vi "Periodic Dot Tracking.vi"() -> ()   [LabVIEW 2012]
panel:
  in  "Delay Time (s)":dbl=1.0
  in  "stop":bool
  out "Gave up?":bool
  out "Y Gauss Amplitude":dbl
  out "Cross Section Y":dbl[](graph)
  out "Cross Section X":dbl[](graph)
  out "Z Position":dbl
  out "Y Position":dbl
  out "X Position":dbl
  in  "Z-track?":bool=TRUE
  in  "Z Pos":dbl=52.1
  in  "Y pos":dbl=35.0
  in  "X Pos":dbl=192.0
  in  "Y Parameters":T1={"Number of Y Steps"=200, "Max Y (V)"=1.0, "Min Y (V)"=-1.0}
  in  "X Parameters":T2={"Number of X Steps"=200, "Max X (V)"=1.0, "Min X (V)"=-1.0}
  in  "RS232 settings":cluster{"Portnumber":i32, "Baudrate":u16}={"Portnumber"=12, "Baudrate"=5} {"Portnumber" items=["COM1", "COM2", "COM3", "COM4", "COM5", "COM6", "COM7", "COM8", "COM9", "COM10", "COM11", "COM12", "COM13", "COM14", "COM15", "COM16", "COM17", "COM18", "COM19", "COM20", "COM21", "COM22", "COM23", "COM24", "COM25", "COM26", "COM27", "COM28", "COM29", "COM30"]; "Baudrate" items=["9600", "14400", "19200", "38400", "57600", "115200"]}
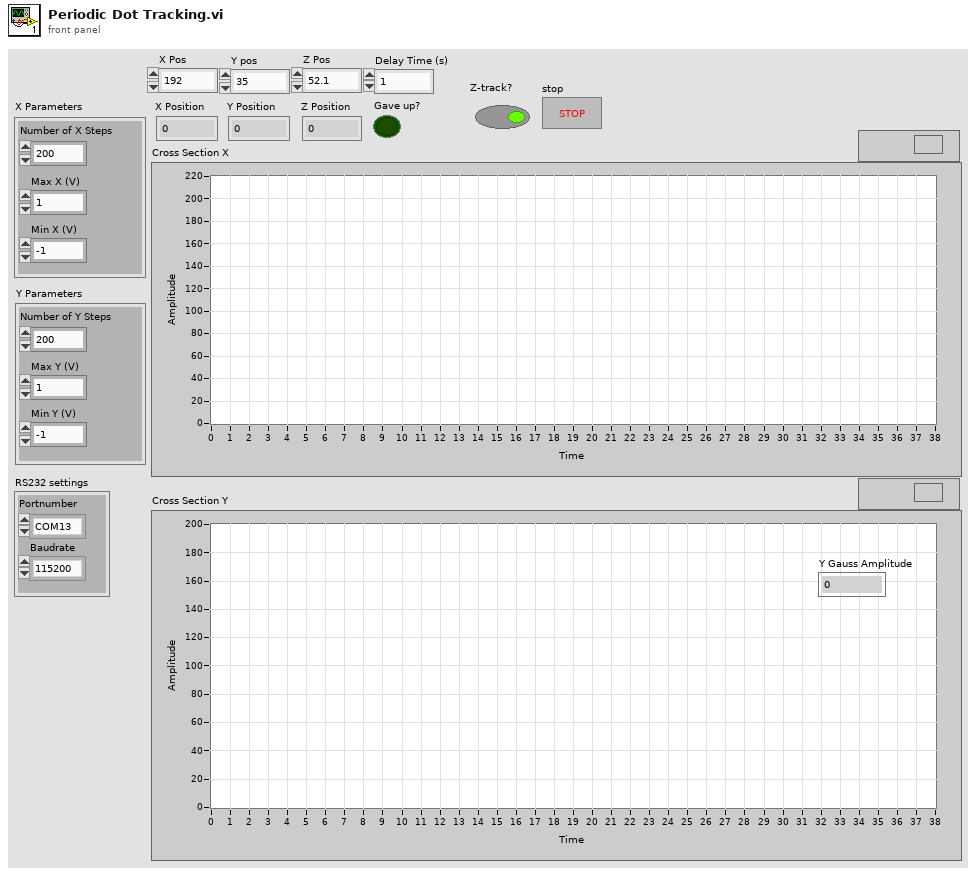
[diagram p1: front panel]
types:
  T1 = cluster{"Number of Y Steps":i32, "Max Y (V)":dbl, "Min Y (V)":dbl}
  T2 = cluster{"Number of X Steps":i32, "Max X (V)":dbl, "Min X (V)":dbl}
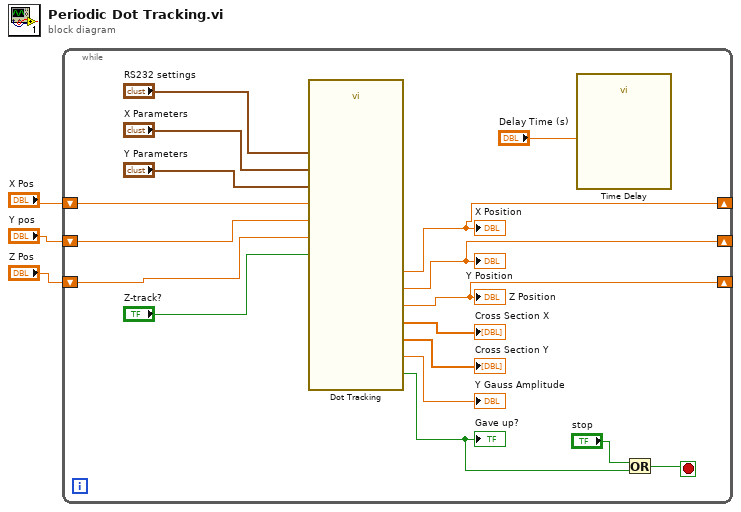
[diagram p0: block diagram]
diagram:
  n1 = while {
    shift-right: [w6] -> _
    shift-left: "X Pos" -> [w9]
    shift-right: [w5] -> _
    shift-left: "Y pos" -> [w8]
    shift-right: [w4] -> _
    shift-left: "Z Pos" -> [w7]
    stop <- w11 stop-if-true
    n2 = call "Dot Tracking.vi"("X Parameters"="X Parameters", "Y Parameters"="Y Parameters", "RS232 settings"="RS232 settings", "X Pos"=w9, "Y pos"=w8, "Z Pos"=w7, "Z-track?"="Z-track?") -> ("X Position"=w6:dbl, "Y Position"=w5:dbl, "Y Gauss Amplitude"=→"Y Gauss Amplitude":dbl, "Z Position"=w4:dbl, "Cross Section X"=→"Cross Section X":dbl[], "Cross Section Y"=→"Cross Section Y":dbl[], "Gave up?"=w12:bool)  [unwired: 2 in]
    "X Position" <- w6
    "Y Position" <- w5
    "Z Position" <- w4
    "Gave up?" <- w12
    n3 = call "Time Delay"("Delay Time (s)"="Delay Time (s)") -> ()  [unwired: 10 in, 1 out]
    n4 = Or(x="stop", y=w12) -> (x .or. y?=w11:bool)
  }
